vi "UIM All Properties.vi"() -> ()   [LabVIEW 2020]
doc: "This example visualizes all different default UIPs handled by UIM. You can modify them using the UI State ring control and see the changes update using the previously captured UIM state."
uses:
  UIM Class/UIM.lvclass
panel:
  in  "XML File":path=path "C:/GitHub/LabVIEW-User-Interface-Manager/Examples/MultiModes.xml" caption="UIM XML Path"
  in  "Table":string[][](table)
  out "Tank":dbl(slide) scale=0.0..10.0
  out "Meter":dbl(knob) scale=0.0..10.0
  in  "Array - String":string[](array[string])
  in  "File Path Control":path
  in  "Listbox":i32(listbox)
  in  "Error In":errorcluster
  out "Waveform Chart":dbl(graph)
  in  "Stop Button 2":bool caption="Boolean"
  in  "Numeric Control":dbl
  in  "Stop Button":bool
  in  "UI State":u16(ring) items=["default", "disabled", "hidden", "position", "size"]
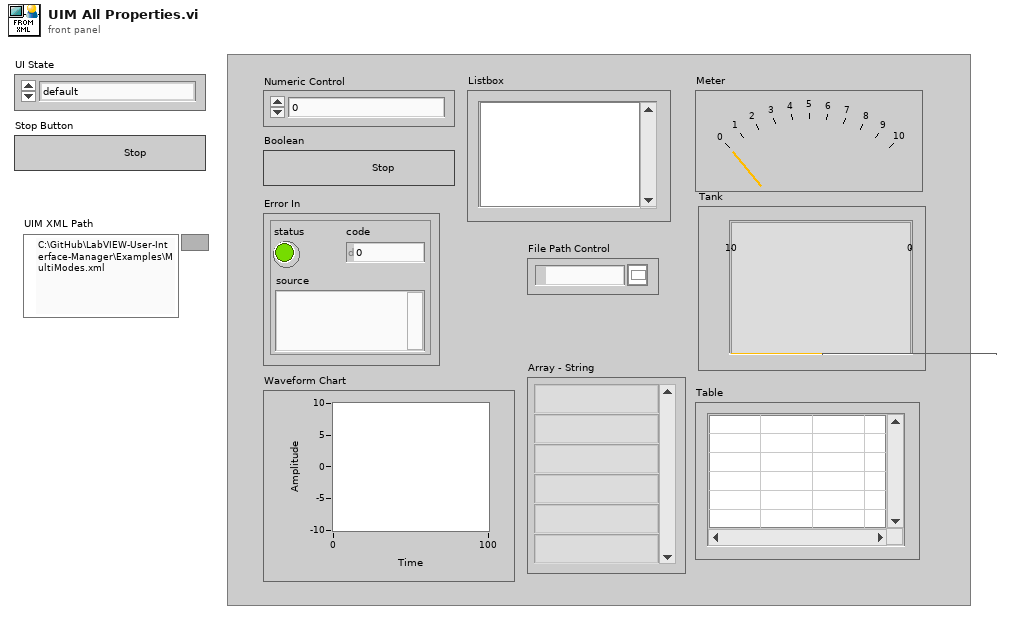
[diagram p1: front panel]
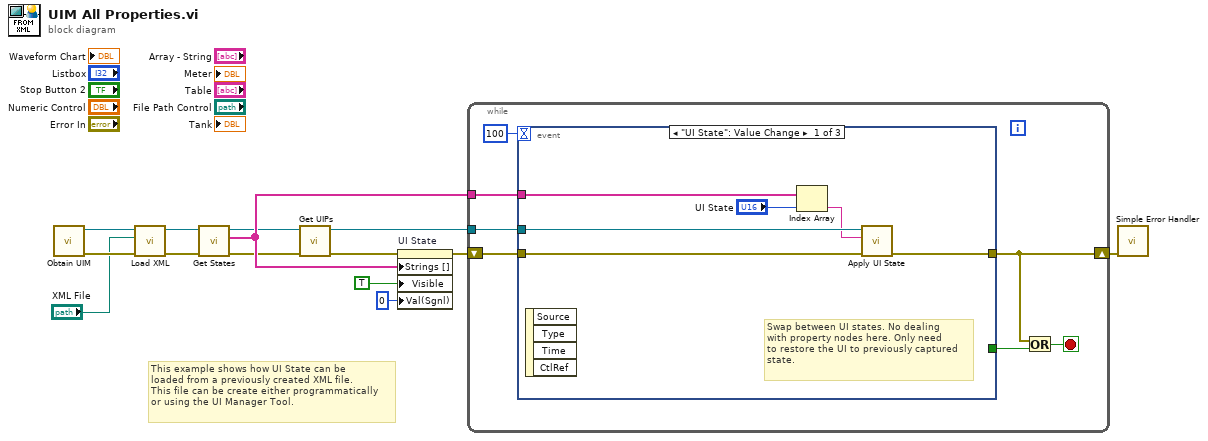
[diagram p0: block diagram]
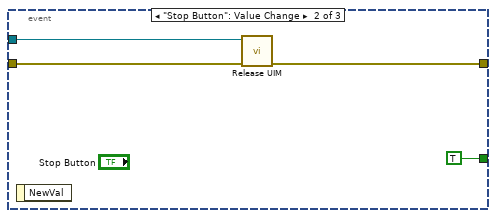
[diagram p2: hidden frame]
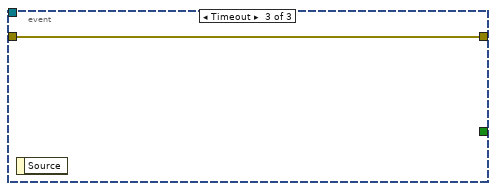
[diagram p3: hidden frame]
diagram:
  # "This example shows how UI State can be\nloaded from a previously created XML file.\nThis file can be create either programmatically\nor using the UI Manager Tool."
  n1 = call "Obtain UIM.vi"() -> ("Error Out"=w8:errorcluster, "UIM Handle"=w11:refnum<data-value>)  [unwired: 10 in]
  n2 = call "Load XML.vi"("Error In"=w8, "XML File"="XML File", "UIM In"=w11) -> ("Error Out"=w9:errorcluster, "UIM Out"=w10:refnum<data-value>)  [unwired: 7 in]
  n3 = call "Get States.vi"("Error In"=w9, "UIM In"=w10) -> ("Error Out"=w3:errorcluster, "States"=w7:string[], "UIM Out"=w4:refnum<data-value>)  [unwired: 7 in]
  n4 = call "Get UIPs.vi"("Error In"=w3, "UIM In"=w4) -> ("Error Out"=w2:errorcluster, "UIM Out"=w1:refnum<data-value>)  [unwired: 6 in, 2 out]
  n5 = property on="UI State" class="Ring (strict)"(error in=w2, "Strings []"=w7, "Visible"=TRUE, "Val(Sgnl)"=u16 0 ("Value (Signaling)")) -> (error out=w14:errorcluster)  [unwired: 1 in, 1 out]
  n6 = while {
    tunnel: w1 -> [w21]
    tunnel: w7 -> [w19]
    shift-right: [w16] -> w6
    shift-left: w14 -> [w20]
    stop <- w17 stop-if-true
    n7 = event shown="[0] \"UI State\": Value Change" {
      selector: _ -> [_ _ _]
      dyn-events: _ -> [_ _ _]
      timeout: 100 -> [_ _ _]
      tunnel: w21 -> [w27 w30 _]
      tunnel: [_ TRUE _] -> w18
      tunnel: w20 -> [w26 w29 w32]
      tunnel: [w25 w28 w32] -> w16
      tunnel: w19 -> [w22 _ _]
      event "UI State": Value Change {
        # "Swap between UI states. No dealing\nwith property nodes here. Only need\nto restore the UI to previously captured\nstate."
        n8 = event-data() -> ()  [unwired: 1 in, 4 out]
        n9 = Index Array(array=w22, index="UI State") -> (element=w23:string)
        n10 = call "Apply UI State.vi"("Error In"=w26, "State Name"=w23, "UIM In"=w27) -> ("Error Out"=w25:errorcluster)  [unwired: 7 in, 1 out]
      }
      event "Stop Button": Value Change {
        n11 = event-data() -> ()  [unwired: 1 in, 1 out]
        n12 = call "Release UIM.vi"("Error In"=w29, "UIM Handle"=w30) -> ("Error Out"=w28:errorcluster)  [unwired: 9 in]
      }
      event Timeout {
        n13 = event-data() -> ()  [unwired: 1 in, 1 out]
      }
    }
    n14 = Or(x=w16, y=w18) -> (x .or. y?=w17:bool)
  }
  n15 = call <vilib>:"Simple Error Handler.vi"("error in (no error)"=w6) -> ()  [unwired: 4 in, 5 out]
